vi "Lockstep Move at Velocity.vi"(7 "Velocity":i32, 8 "error in (no error)":errorcluster, 9 "Device Number":string, 10 "Lockstep Group (1)":u8=1, 11 "VISA resource name":refnum<visa-resource-name>) -> (0 "error out":errorcluster, 3 "VISA resource name out":refnum<visa-resource-name>)   [LabVIEW 2013, in "Zaber A Series.lvlib"]
doc: "Moves a lockstep group at a specified velocity. Velocity is specified in native device speed units; check your device manual for the conversion factor or use the Conver Velocity Units to Device Units VI.\n\nConstant velocity movement stops when the stage reaches the end of its travel, a stop command is sent, or a new movement command is sent.\n\nThis VI requires that the Initialize VI has been called with the same serial port and that the lockstep group has already been enabled. \n\nNote: See the Device Lookup control for the microstep size of your model, or check on the product specifications page for the product on www.zaber.com."
uses:
  Zaber A Series.lvlib
  Private/All Commands.ctl
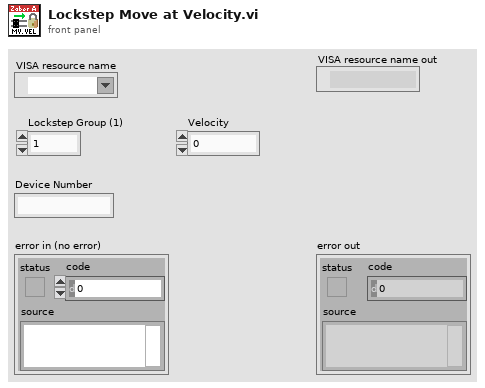
[diagram p1: front panel]
types:
  T1 = typedef "Zaber A Series.lvlib/All Commands.ctl" = string
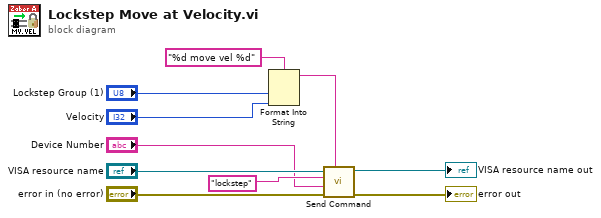
[diagram p0: block diagram]
diagram:
  n1 = Format Into String(format string="%d move vel %d", "Lockstep Group (1)", "Velocity") -> (resulting string=w5:string)  [unwired: 2 in, 1 out]
  n2 = call "Send Command.vi"("Data"=w5, "error in (no error)"="error in (no error)", "Device and Axis"="Device Number", "Command"=T1 "lockstep" ("Complete Command List"), "VISA resource name"="VISA resource name") -> ("error out"=→"error out":errorcluster, "VISA resource name out"=→"VISA resource name out":refnum<visa-resource-name>)  [unwired: 1 in, 4 out]
